vi "Shock Detect.vi"(4 "Zero":bool, 6 "Period (sec)":dbl=1.0, 9 "Threshold (mG)":dbl=50.0, 10 "Ref (mG)":dbl, 11 "Acc X,Y,Z":cluster{"X Acc":dbl, "Y Acc":dbl, "Z Acc":dbl}) -> (0 "Shock Level":dbl=2187.509013360497, 1 "Shock Period":bool, 2 "Shock":bool, 3 "Acc Vector":dbl=11.874342087037917)   [LabVIEW 2017]
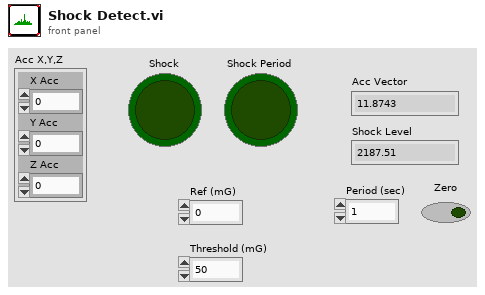
[diagram p1: front panel]
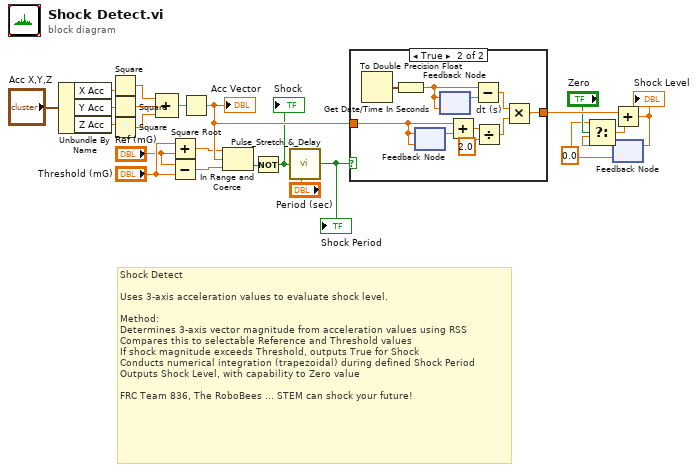
[diagram p0: block diagram]
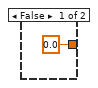
[diagram p2: hidden frame]
diagram:
  w16 = 0.0
  # "Shock Detect\n\nUses 3-axis acceleration values to evaluate shock level.\n\nMethod:\nDetermines 3-axis vector magnitude from acceleration values using RSS\nCompares this to selectable Reference and Threshold values\nIf shock magnitude exceeds Threshold, outputs True for Shock\nConducts numerical integration (trapezoidal) during defined Shock Period\nOutputs Shock Level, with capability to Zero value\n\nFRC Team 836, The RoboBees ... STEM can shock your future!"
  n1 = Unbundle By Name("Acc X,Y,Z") -> ("X Acc"=w20:dbl, "Y Acc"=w21:dbl, "Z Acc"=w22:dbl)
  n2 = Square(x=w20) -> (x^2=w2:dbl)
  n3 = Square(x=w21) -> (x^2=w3:dbl)
  n4 = Square(x=w22) -> (x^2=w4:dbl)
  n5 = Compound Arithmetic op=ADD(w2, w3, w4) -> (w5:dbl)
  n6 = Add(x="Threshold (mG)", y="Ref (mG)") -> (x+y=w7:dbl)
  n7 = Subtract(x="Ref (mG)", y="Threshold (mG)") -> (x-y=w6:dbl)
  n8 = Square Root(x=w5) -> (sqrt(x)=w12:dbl)
  "Acc Vector" <- w12
  n9 = In Range and Coerce(upper limit=w7, x=w12, lower limit=w6) -> (In Range?=w1:bool)  [unwired: 1 out]
  n10 = Not(x=w1) -> (.not. x?=w11:bool)
  "Shock" <- w11
  n11 = call <userlib>:"Pulse_Stretch_&_Delay.vi"("In"=w11, "Width (sec)"="Period (sec)") -> ("Out"=w23:bool)  [unwired: 3 in]
  "Shock Period" <- w23
  n12 = case shown="True" w23 {
    tunnel: w12 -> [_ w27]
    tunnel: [0.0 w25] -> w18
    frame False {
    }
    frame True {
      n13 = Get Date/Time In Seconds() -> (seconds since 1Jan1904=w34:timestamp)
      n14 = To Double Precision Float(number=w34) -> (double precision float=w26:dbl)
      n15 = feedback #1(w27) -> (w30:dbl)
      n16 = feedback-in #1(w27) -> ()
      n17 = feedback #2(w26) -> (w28:dbl)
      n18 = feedback-in #2(w26) -> ()
      n19 = Add(x=w27, y=w30) -> (x+y=w29:dbl)
      n20 = Subtract "dt (s)"(x=w26, y=w28) -> (x-y=w32:dbl)
      n21 = Divide(x=w29, y=2.0) -> (x/y=w33:dbl)
      n22 = Multiply(x=w32, y=w33) -> (x*y=w25:dbl)
    }
  }
  n23 = feedback #3(w16) -> (w15:dbl)
  n24 = Select(t=w16, s="Zero", f=w15) -> (s? t:f=w14:dbl)
  n25 = Add(x=w18, y=w14) -> (x+y=w13:dbl)
  "Shock Level" <- w13
  n26 = feedback-in #3(w13) -> ()
